vi "OCR_Test_Right_3_Digit.vi"(0 "x Top":dbl, 1 "y Top":dbl, 5 "x Center":dbl, 7 "Image in":T1(plugin-control), 9 "y Center":dbl, 11 "x Bottom":dbl, 12 "y Bottom":dbl, 14 "error in":errorcluster) -> (3 "Read Top":string caption="Read String", 6 "Read Center":string, 10 "error out":errorcluster, 15 "Read bottom":string)   [LabVIEW 2019]
uses:
  <vilib>/vision/NI_Vision_Development_Module.lvlib
panel:
  in  "Training File Path":path=path "D:/Focusing Station/Sub VIs/OCR_Test_R_C.abc"
  out "Image":T1(plugin-control)
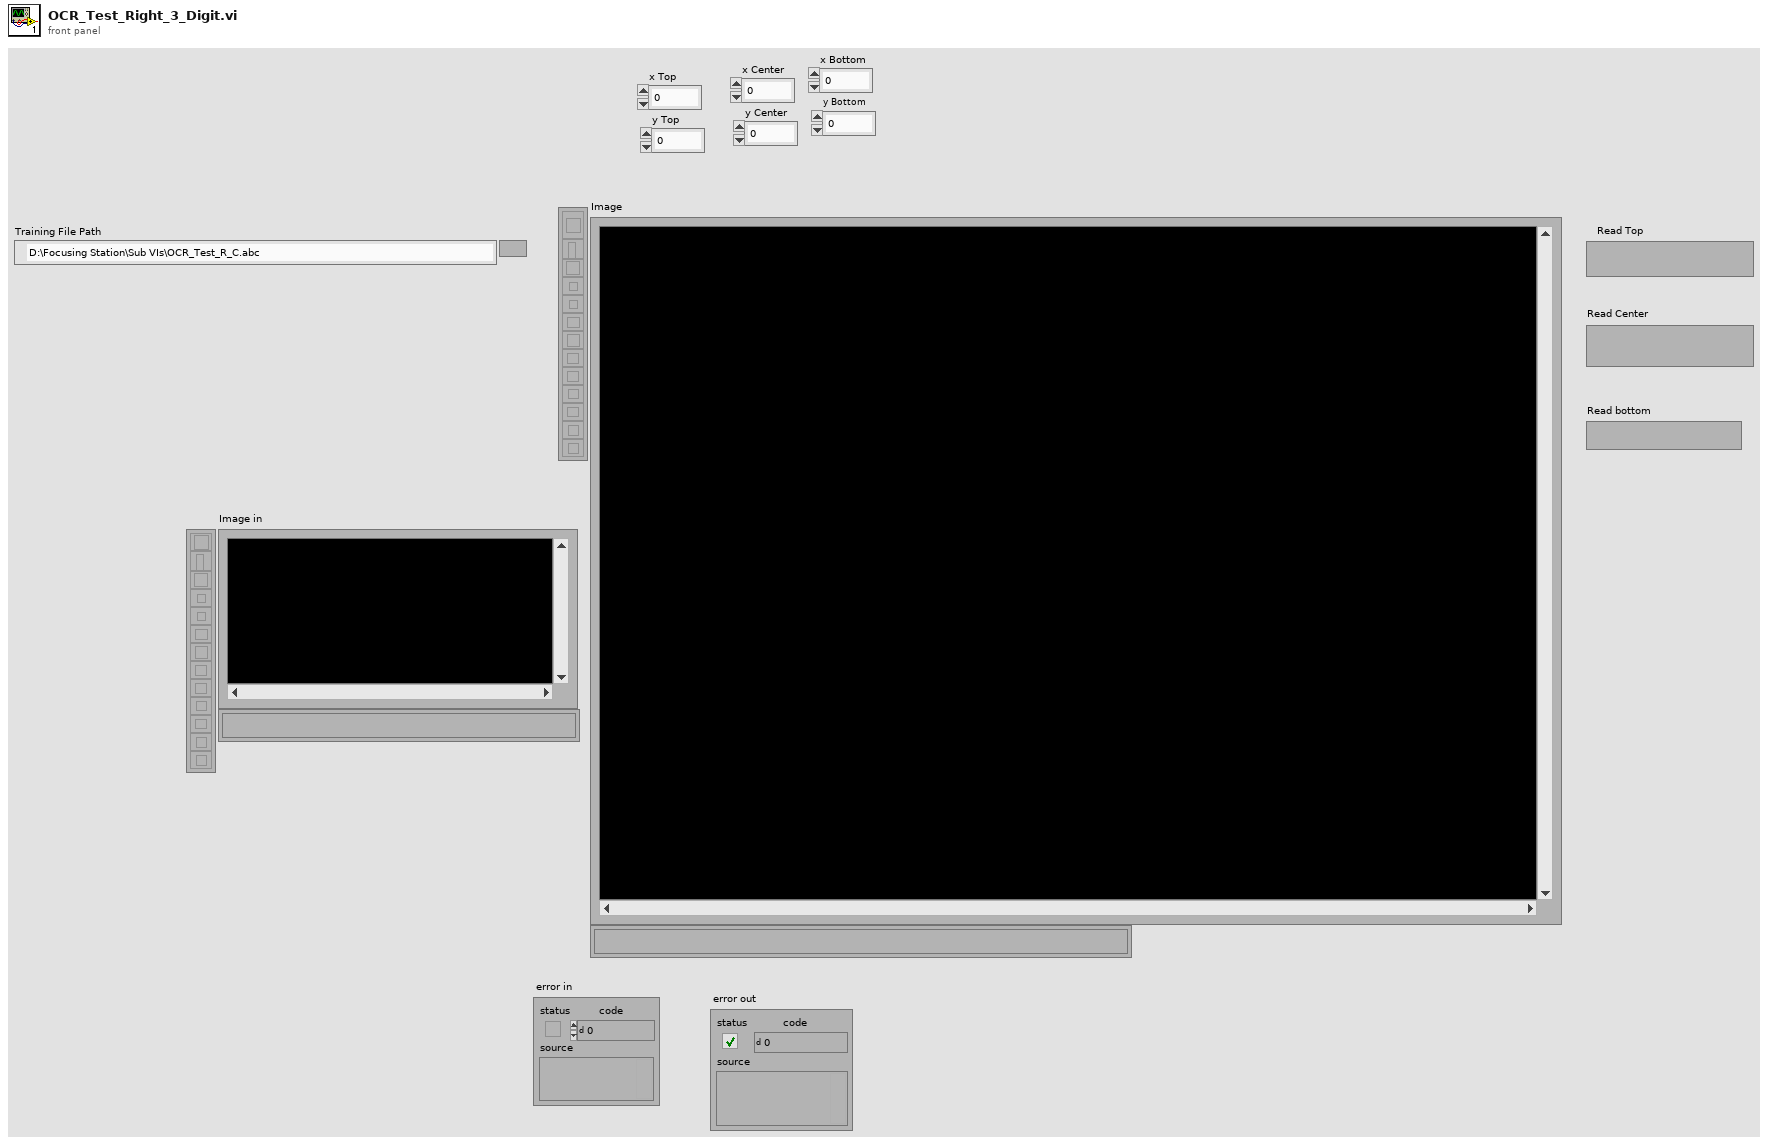
[diagram p1: front panel]
types:
  T1 = typedef "IMAQ Image.ctl" = refnum<image>
  T2 = typedef "IMAQ Rectangle" = cluster{"Left":i32, "Top":i32, "Right":i32, "Bottom":i32, "Rotation":dbl}
  T3 = typedef "IMAQ OCR Session.ctl" = refnum<k1>
  T4 = typedef "ROI Descriptor" = cluster{"Global Rectangle":i32[], "Contours":cluster{"ID":enum32{"External", "Internal"}, "Type":u32, "Coordinates":i32[]}[]}
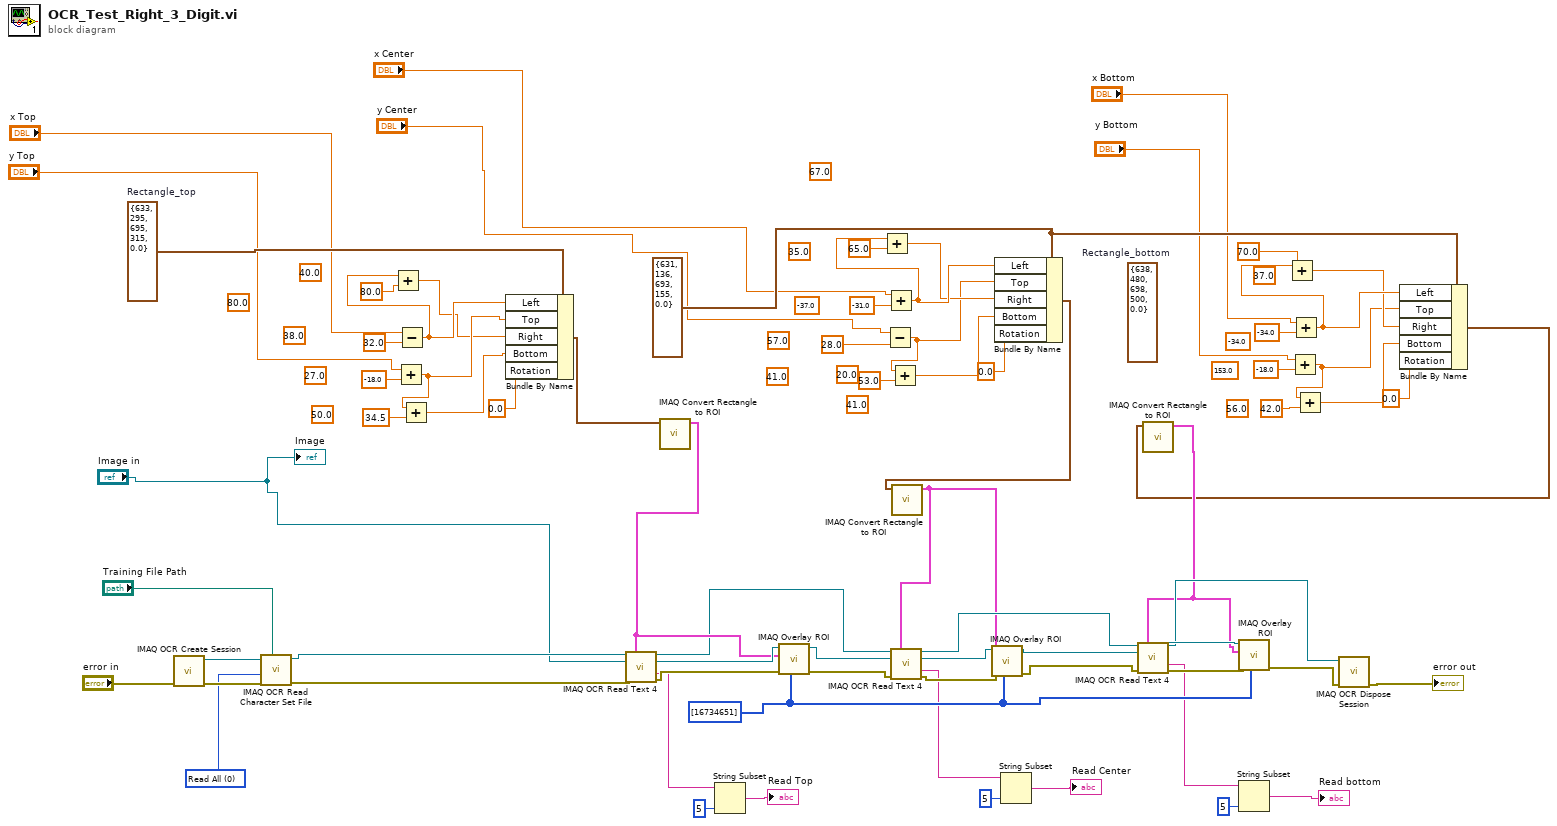
[diagram p0: block diagram]
diagram:
  (unwired) sgl 56.0 ("y")
  (unwired) sgl -34.0 ("y")
  (unwired) sgl 41.0 ("y")
  (unwired) sgl 40.0 ("y")
  (unwired) sgl 35.0 ("y")
  (unwired) sgl -37.0 ("y")
  (unwired) sgl 67.0 ("y")
  (unwired) sgl 50.0 ("y")
  (unwired) sgl 27.0 ("y")
  (unwired) sgl 38.0 ("y")
  (unwired) sgl 153.0 ("y")
  (unwired) sgl 57.0 ("y")
  (unwired) sgl 80.0 ("y")
  (unwired) sgl 37.0 ("y")
  (unwired) sgl 41.0 ("y")
  (unwired) sgl 20.0 ("y")
  (unwired) T2 {"Left"=638, "Top"=480, "Right"=698, "Bottom"=500, "Rotation"=0.0}  # Rectangle_bottom
  w33 = T2 {"Left"=631, "Top"=136, "Right"=693, "Bottom"=155, "Rotation"=0.0}
  w67 = 0 items=["Read All", "Read Character Set Only", "Read Properties Only"] ("Read Options")
  w27 = T2 {"Left"=633, "Top"=295, "Right"=695, "Bottom"=315, "Rotation"=0.0}  # Rectangle_top
  w52 = u32[] [16734651] ("Colors (Green)")
  n1 = call "IMAQ OCR Create Session"("error in (no error)"="error in") -> ("error out"=w73:errorcluster, "IMAQ OCR Session"=w74:T3)  [unwired: 9 in]
  n2 = call "IMAQ OCR Read Character Set File"("File Path"="Training File Path", "error in (no error)"=w73, "Read Options"=w67, "IMAQ OCR Session"=w74) -> ("error out"=w70:errorcluster, "IMAQ OCR Session (dup)"=w71:T3)  [unwired: 5 in, 1 out]
  n3 = Add(x="y Top", y=sgl -18.0) -> (x+y=w25:dbl)
  n4 = Subtract(x="x Top", y=sgl 32.0) -> (x-y=w26:dbl)
  n5 = Add(x=w26, y=sgl 80.0) -> (x+y=w24:dbl)
  n6 = Add(x=w25, y=sgl 34.5) -> (x+y=w23:dbl)
  n7 = Bundle By Name(cluster=w27, "Left"=w26, "Top"=w25, "Right"=w24, "Bottom"=w23, "Rotation"=0.0) -> (w22:T2)
  n8 = call "IMAQ Convert Rectangle to ROI"("Rectangle"=w22) -> ("ROI Descriptor"=w66:T4)  [unwired: 8 in, 1 out]
  n9 = call "IMAQ OCR Read Text 4"("IMAQ OCR Session"=w71, "ROI Descriptor"=w66, "Image"="Image in", "error in (no error)"=w70) -> ("IMAQ OCR Session (dup)"=w62:T3, "Image (dup)"=w68:T1, "Read String"=w9:string, "error out"=w69:errorcluster)  [unwired: 5 in, 3 out]
  n10 = String Subset(string=w9, length (rest)=5 ("length (rest)")) -> (substring=→"Read Top":string)  [unwired: 1 in]
  n11 = call "IMAQ Overlay ROI"("Colors (Green)"=w52, "error in (no error)"=w69, "ROI Descriptor"=w66, "Image"=w68) -> ("error out"=w60:errorcluster, "Image Out"=w61:T1)  [unwired: 2 in, 4 out]
  n12 = Subtract(x="y Center", y=sgl 28.0) -> (x-y=w44:dbl)
  n13 = Add(x="x Center", y=sgl -31.0) -> (x+y=w46:dbl)
  n14 = Add(x=w46, y=sgl 65.0) -> (x+y=w45:dbl)
  n15 = Add(x=w44, y=sgl 53.0) -> (x+y=w43:dbl)
  n16 = Bundle By Name(cluster=w33, "Left"=w46, "Top"=w44, "Right"=w45, "Bottom"=w43, "Rotation"=0.0) -> (w42:T2)
  n17 = call "IMAQ Convert Rectangle to ROI"("Rectangle"=w42) -> ("ROI Descriptor"=w50:T4)  [unwired: 8 in, 1 out]
  n18 = call "IMAQ OCR Read Text 4"("IMAQ OCR Session"=w62, "ROI Descriptor"=w50, "Image"=w61, "error in (no error)"=w60) -> ("IMAQ OCR Session (dup)"=w55:T3, "Image (dup)"=w64:T1, "Read String"=w4:string, "error out"=w63:errorcluster)  [unwired: 5 in, 3 out]
  n19 = call "IMAQ Overlay ROI"("Colors (Green)"=w52, "error in (no error)"=w63, "ROI Descriptor"=w50, "Image"=w64) -> ("error out"=w56:errorcluster, "Image Out"=w57:T1)  [unwired: 2 in, 4 out]
  n20 = String Subset(string=w4, length (rest)=5 ("length (rest)")) -> (substring=→"Read Center":string)  [unwired: 1 in]
  n21 = Add(x="y Bottom", y=sgl -18.0) -> (x+y=w35:dbl)
  n22 = Add(x="x Bottom", y=sgl -34.0) -> (x+y=w37:dbl)
  n23 = Add(x=w37, y=sgl 70.0) -> (x+y=w36:dbl)
  n24 = Add(x=w35, y=sgl 42.0) -> (x+y=w34:dbl)
  n25 = Bundle By Name(cluster=w33, "Left"=w37, "Top"=w35, "Right"=w36, "Bottom"=w34, "Rotation"=0.0) -> (w32:T2)
  n26 = call "IMAQ Convert Rectangle to ROI"("Rectangle"=w32) -> ("ROI Descriptor"=w51:T4)  [unwired: 8 in, 1 out]
  n27 = call "IMAQ OCR Read Text 4"("IMAQ OCR Session"=w55, "ROI Descriptor"=w51, "Image"=w57, "error in (no error)"=w56) -> ("IMAQ OCR Session (dup)"=w54:T3, "Image (dup)"=w58:T1, "Read String"=w3:string, "error out"=w59:errorcluster)  [unwired: 5 in, 3 out]
  n28 = call "IMAQ Overlay ROI"("Colors (Green)"=w52, "error in (no error)"=w59, "ROI Descriptor"=w51, "Image"=w58) -> ("error out"=w53:errorcluster)  [unwired: 2 in, 5 out]
  n29 = String Subset(string=w3, length (rest)=5 ("length (rest)")) -> (substring=→"Read bottom":string)  [unwired: 1 in]
  n30 = call "IMAQ OCR Dispose Session"("error in (no error)"=w53, "IMAQ OCR Session"=w54) -> ("error out"=→"error out":errorcluster)  [unwired: 9 in]
  "Image" <- "Image in"
